vi "get power.vi"(8 "error in (no error)":errorcluster, 11 "Cobolt in":refnum<class "Cobolt.lvclass">) -> (0 "error out":errorcluster, 3 "Cobolt out":refnum<class "Cobolt.lvclass">)   [LabVIEW 2012, in "Cobolt.lvclass"]
uses:
  Cobolt.lvclass
  CoboltLaserDrivers_Public_LV2012/CoboltLaser_Controls/ExpectedResponseType.ctl
  Cobolt.lvclass/Cobolt.ctl
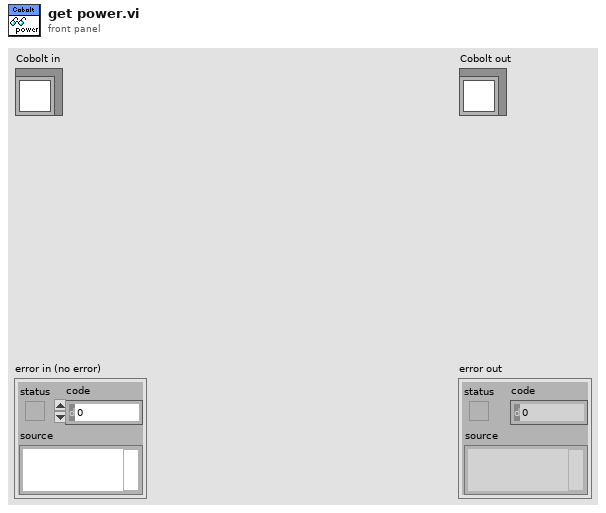
[diagram p1: front panel]
types:
  T1 = typedef "Cobolt.lvclass/ExpectedResponseType.ctl" = u16
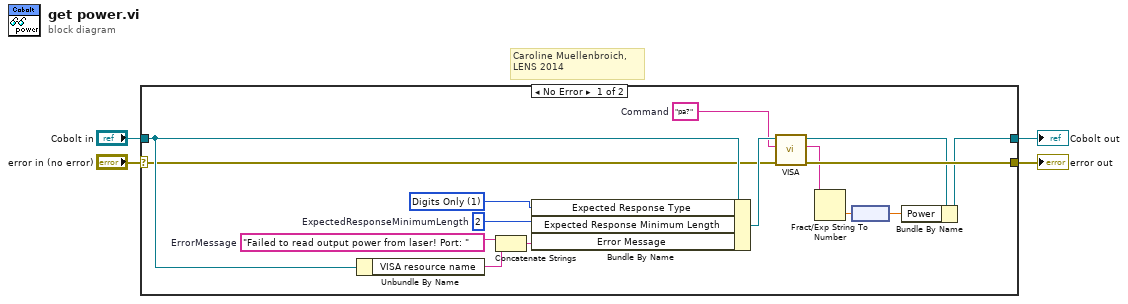
[diagram p0: block diagram]
diagram:
  # "Caroline Muellenbroich, \nLENS 2014"
  n1 = case shown="No Error" "error in (no error)" {
    selector: "error in (no error)" -> [w12 w21]
    tunnel: [w11 w21] -> w3
    tunnel: [w7 w20] -> w1
    tunnel: "Cobolt in" -> [w13 w20]
    frame No Error {
      w19 = T1 1 items=["Any", "Digits Only", "Non-Digits Only"] ("ExpectedResponseType")
      w15 = 2  # ExpectedResponseMinimumLength
      w17 = "Failed to read output power from laser! Port: "  # ErrorMessage
      w10 = "pa?"  # Command
      n2 = Unbundle By Name(w13) -> ("VISA resource name"=w16:string)
      n3 = Concatenate Strings(w17, w16) -> (w18:string)
      n4 = Bundle By Name(cluster=w13, "Expected Response Type"=w19, "Expected Response Minimum Length"=w15, "Error Message"=w18) -> (w14:refnum<class "Cobolt.lvclass">)
      n5 = call-dynamic "VISA.vi"("error in (no error)"=w12, "string to write"=w10, "Cobolt in"=w14) -> ("error out"=w11:errorcluster, "buffer out"=w9:string, "Cobolt out"=w8:refnum<class "Cobolt.lvclass">)  [unwired: 6 in]
      n6 = Fract/Exp String To Number(string=w9) -> (number=w6:dbl)  [unwired: 3 in, 1 out]
      n7 = node(w6) -> (w5:dbl[unit])
      n8 = Bundle By Name(cluster=w8, "Power"=w5) -> (w7:refnum<class "Cobolt.lvclass">)
    }
    frame Error {
    }
  }
  "error out" <- w3
  "Cobolt out" <- w1
